vi "CoboltLaser_LaserOff.vi"(0 "ComPort":refnum<visa-resource-name>, 3 "GenerateError":bool=TRUE, 7 "error in (no error)":errorcluster) -> (20 "ComPortOut":refnum<visa-resource-name>, 21 "Response":string, 23 "ResponseOK":bool, 27 "error out":errorcluster)   [LabVIEW 2019]
doc: "Use this template to build a VI to use as a subVI."
uses:
  <userlib>/CoboltLaser/CoboltLaser_Controls/ExpectedResponseType.ctl
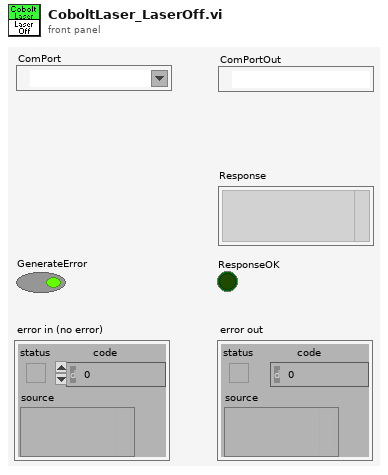
[diagram p1: front panel]
types:
  T1 = typedef "ExpectedResponseType.ctl" = enum16{"Any", "Digits Only", "Non-Digits Only"}
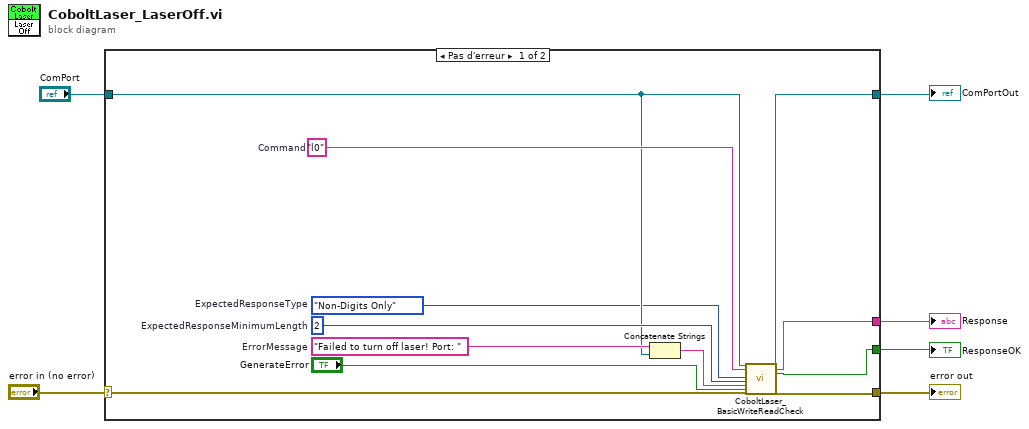
[diagram p0: block diagram]
diagram:
  n1 = case shown="Pas d'erreur" "error in (no error)" {
    selector: "error in (no error)" -> [w18 w20]
    tunnel: [w17 w20] -> w5
    tunnel: "ComPort" -> [w11 w19]
    tunnel: [w10 w19] -> w3
    tunnel: [w9 _] -> w2
    tunnel: [w8 _] -> w1
    frame No Error {
      w7 = ExpectedResponseType."Non-Digits Only"  # ExpectedResponseType
      w16 = 2  # ExpectedResponseMinimumLength
      w14 = "Failed to turn off laser! Port: "  # ErrorMessage
      w12 = "l0"  # Command
      n2 = Concatenate Strings(w14, w11) -> (w13:string)
      n3 = call <userlib>:"CoboltLaser_BasicWriteReadCheck.vi"("ComPort"=w11, "Command"=w12, "ExpectedResponseType"=w7, "ExpectedResponseMinimumLength"=w16, "ErrorMessage"=w13, "GenerateError"="GenerateError", "error in (no error)"=w18) -> ("ComPortOut"=w10:refnum<visa-resource-name>, "Response"=w9:string, "ResponseOK"=w8:bool, "error out"=w17:errorcluster)  [unwired: 17 in]
    }
    frame Error {
    }
  }
  "error out" <- w5
  "Response" <- w2
  "ComPortOut" <- w3
  "ResponseOK" <- w1
